vi "Write step.vi"(8 "error in (no error)":errorcluster, 10 "step":dbl, 11 "Optics in":refnum<class "Optics.lvclass">) -> (0 "error out":errorcluster, 3 "Optics out":refnum<class "Optics.lvclass">)   [LabVIEW 2018, in "Optics.lvclass"]
uses:
  Optics.lvclass
  Optics.lvclass/Optics.ctl
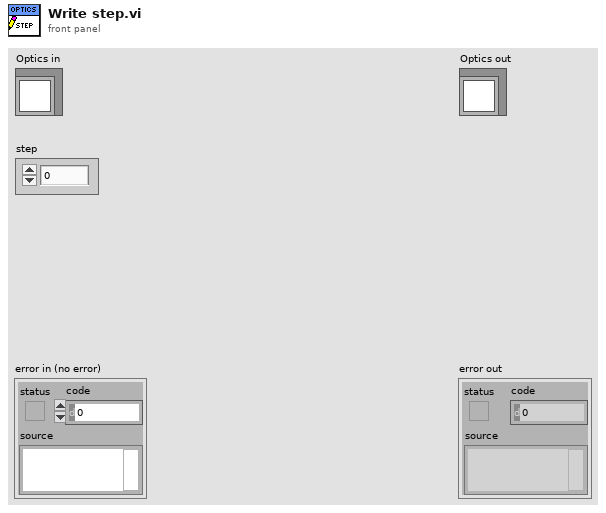
[diagram p1: front panel]
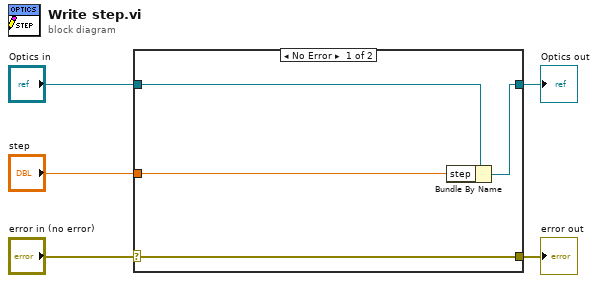
[diagram p0: block diagram]
diagram:
  n1 = case shown="No Error" "error in (no error)" {
    selector: "error in (no error)" -> [w9 w10]
    tunnel: [w9 w10] -> w4
    tunnel: [w7 w11] -> w2
    tunnel: "Optics in" -> [w8 w11]
    tunnel: "step" -> [w6 _]
    frame No Error {
      n2 = Bundle By Name(cluster=w8, "step"=w6) -> (w7:refnum<class "Optics.lvclass">)
    }
    frame Error {
    }
  }
  "error out" <- w4
  "Optics out" <- w2
